vi "Functional Global Variable.vi"(9 "Action":T1, 11 "Initialize to":i32) -> (3 "Result":i32)   [LabVIEW 2016]
uses:
  Action Items.ctl
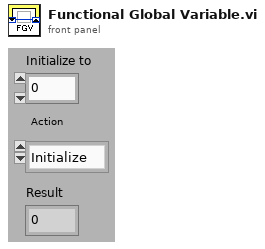
[diagram p1: front panel]
types:
  T1 = typedef "Action Items.ctl" = enum16{"Initialize", "Get", "Increment"}
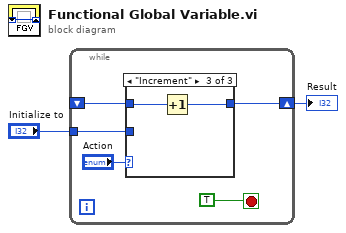
[diagram p0: block diagram]
diagram:
  n1 = while {
    shift-right: [w7] -> w1
    shift-left: _ -> [w6]
    tunnel: "Initialize to" -> [w3]
    stop <- TRUE ("stop") stop-if-true
    n2 = case shown="\"Increment\"" "Action" {
      tunnel: [w8 w9 w10] -> w7
      tunnel: w6 -> [_ w9 w11]
      tunnel: w3 -> [w8 _ _]
      frame "Initialize" {
      }
      frame "Get" {
      }
      frame "Increment" {
        n3 = Increment(x=w11) -> (x+1=w10:i32)
      }
    }
  }
  "Result" <- w1
